vi "ReducePixels(SubVI).vi"(10 "Array in":dbl[][](array[numeric]), 11 "length":i32) -> (3 "Array out":dbl[][](array[numeric]))   [LabVIEW 2014]
uses:
  <vilib>/Analysis/baseanly.llb/Mean (DBL).vi
  <vilib>/Analysis/NI_AALBase.lvlib
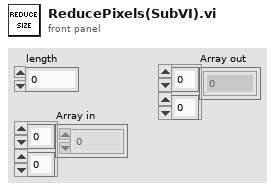
[diagram p1: front panel]
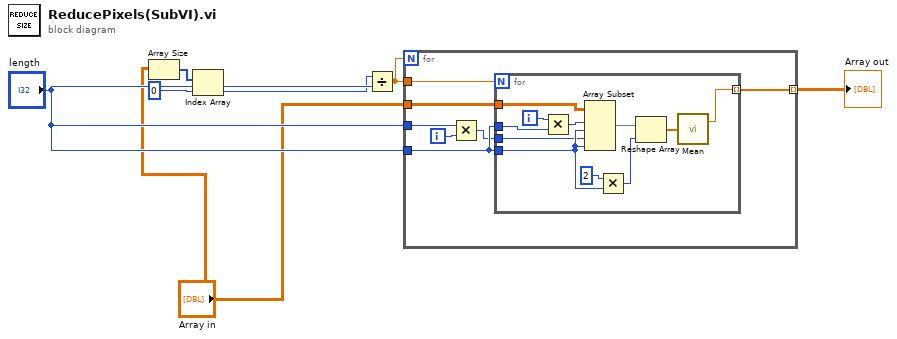
[diagram p0: block diagram]
diagram:
  n1 = Array Size(array="Array in") -> (size(s)=w2:i32[])
  n2 = Index Array(array=w2, index=0) -> (element=w4:i32)
  n3 = Divide(x=w4, y="length") -> (x/y=w6:dbl)
  n4 = for {
    N: w6 -> [_]
    tunnel: "Array in" -> [w14]
    tunnel: w6 -> [w13]
    tunnel: "length" -> [w12]
    tunnel: "length" -> [w9]
    tunnel: [w8] -> w7 mode=indexing
    i -> [w11]
    n5 = Multiply(x=w9, y=w11) -> (x*y=w10:i32)
    n6 = for {
      N: w13 -> [_]
      tunnel: w14 -> [w25]
      tunnel: w12 -> [w23]
      tunnel: w12 -> [w18]
      tunnel: w10 -> [w16]
      tunnel: [w15] -> w8 mode=indexing
      i -> [w20]
      n7 = Multiply(x=w20, y=w18) -> (x*y=w19:i32)
      n8 = Array Subset(array=w25, index (row)=w19, length (row)=w23, index (col)=w16, length (col)=w23) -> (w24:dbl[][])
      n9 = Multiply(x=2, y=w23) -> (x*y=w22:i32)
      n10 = Reshape Array(w24, w22) -> (w17:dbl[])
      n11 = call-poly <vilib>:"Mean.vi"("X"=w17) -> ("mean"=w15:dbl)  [unwired: 1 out]
    }
  }
  "Array out" <- w7
